vi "readVNAssss.vi"() -> ()   [LabVIEW 2020]
uses:
  <vilib>/Utility/file.llb/Read Delimited Spreadsheet (DBL).vi
  <vilib>/Utility/file.llb/Write Delimited Spreadsheet (string).vi
panel:
  out "all rows 2":dbl[][](array[numeric])
  out "text 2":string
  out "after substring 2":string
  out "string array 4":string[](array[string])
  out "string array 3":string[][](array[string])
  out "string array 2":string[][](array[string])
  out "string array":string[](array[string])
  out "after substring":string
  out "text":string
  out "all rows":dbl[][](array[numeric])
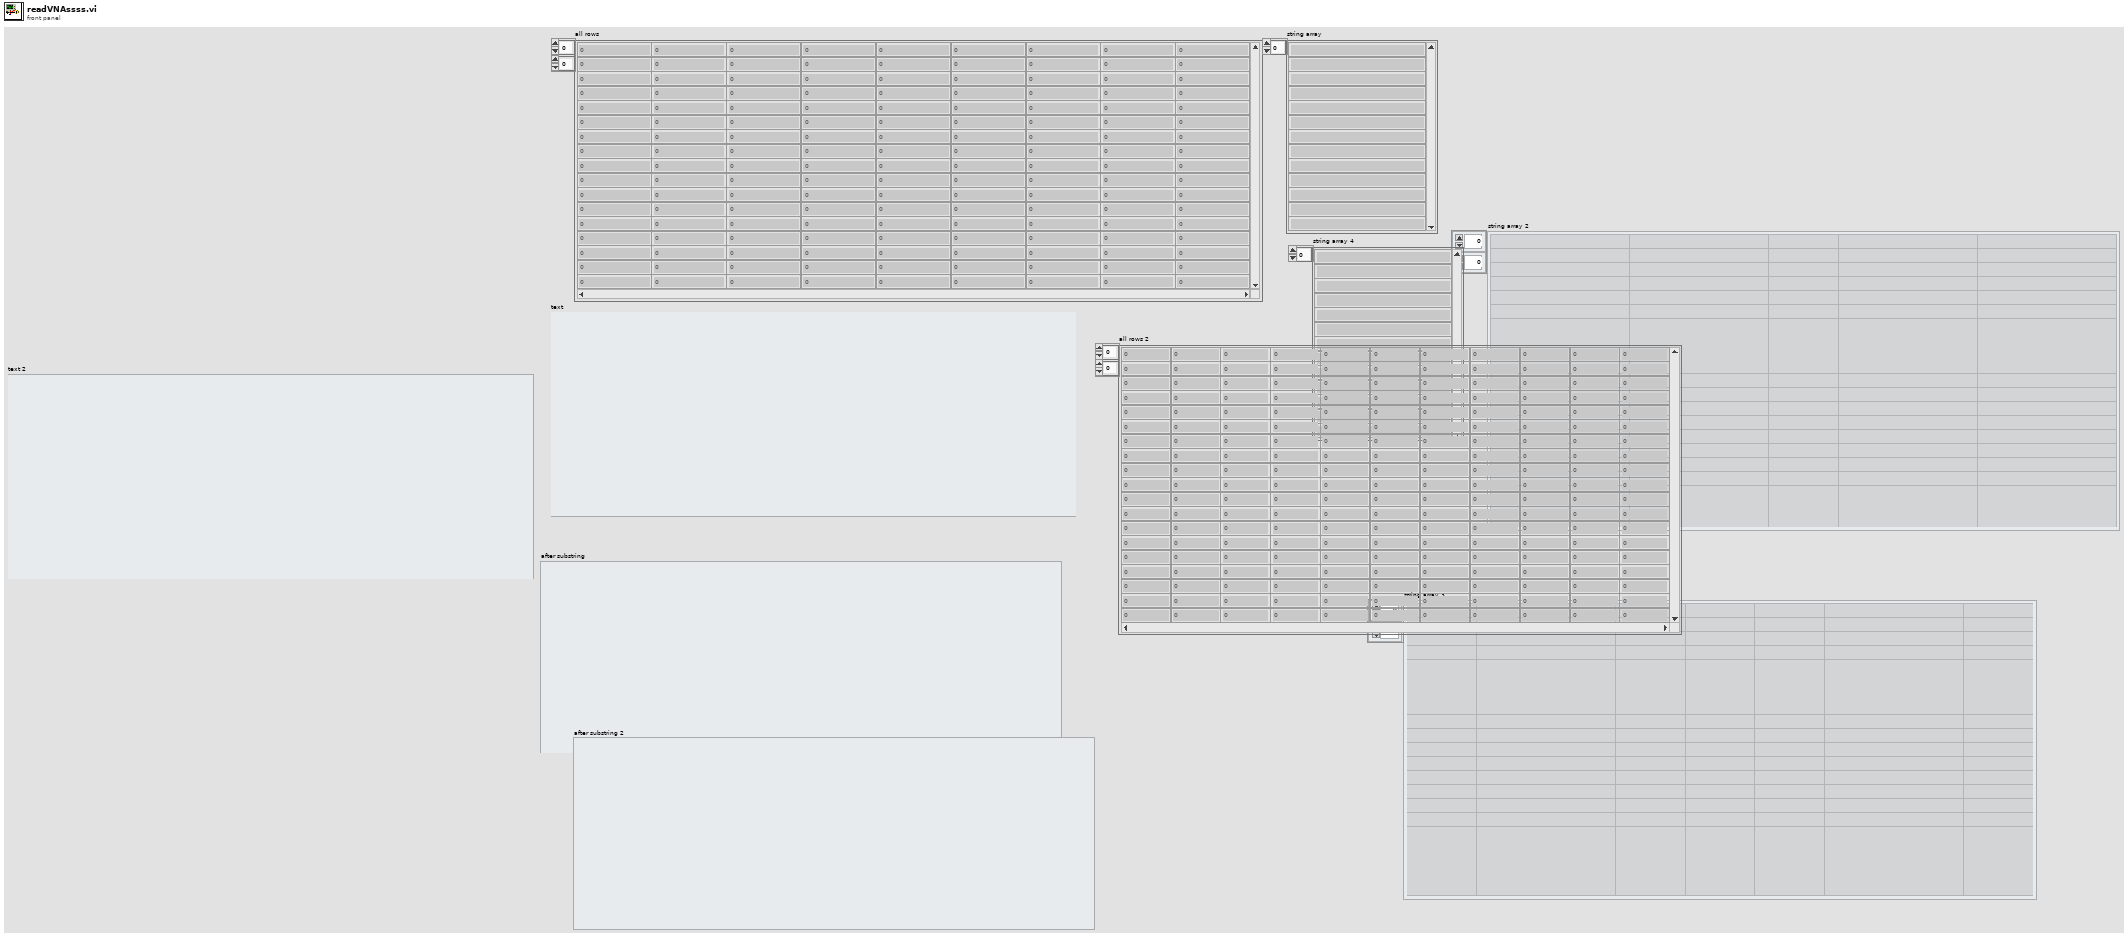
[diagram p1: front panel]
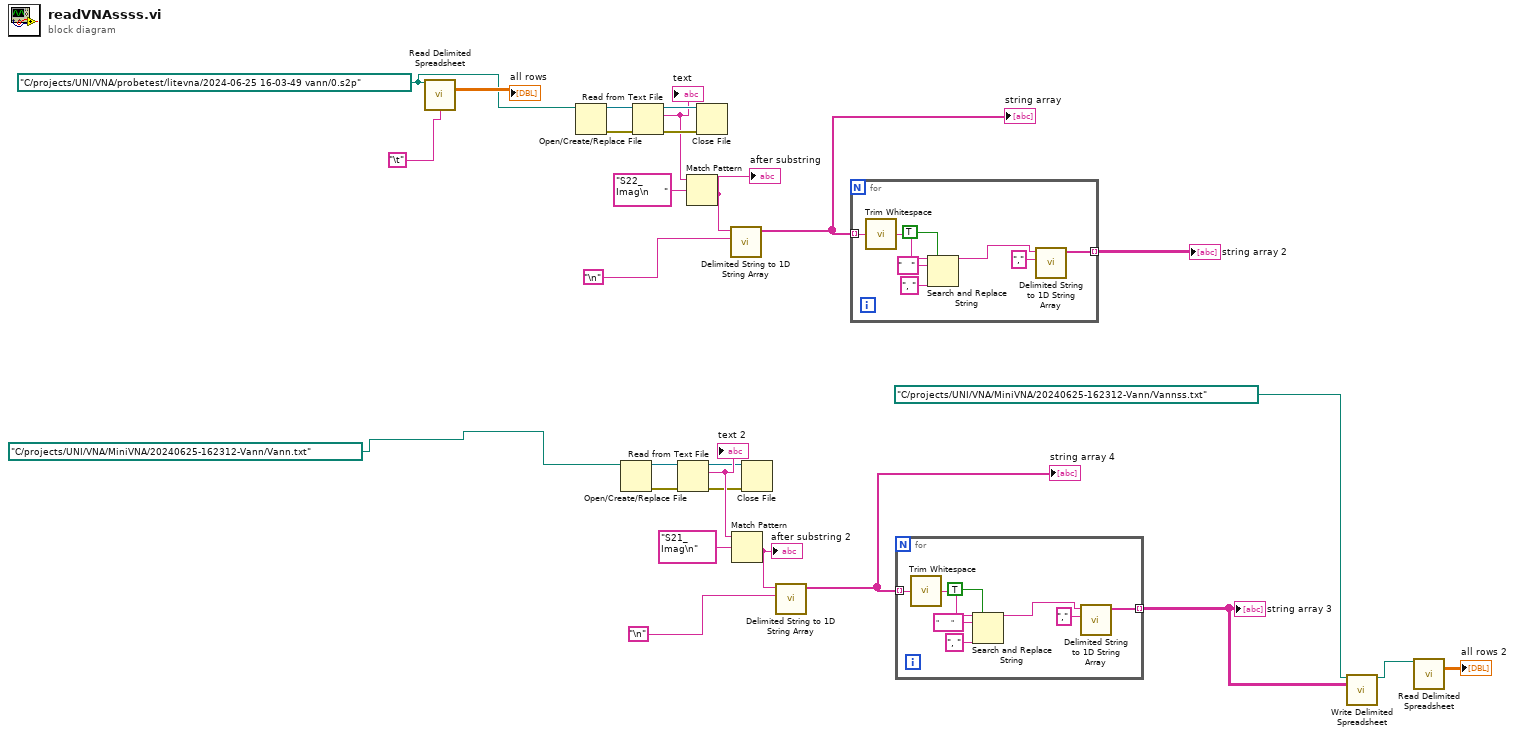
[diagram p0: block diagram]
diagram:
  w21 = path "C:/projects/UNI/VNA/probetest/litevna/2024-06-25 16-03-49 vann/0.s2p" ("file path (dialog if empty)")
  n1 = call-poly <vilib>:"Read Delimited Spreadsheet.vi"("file path (dialog if empty)"=w21, "delimiter (\\t)"="\t") -> ("all rows"=→"all rows":dbl[][])  [unwired: 8 in, 5 out]
  n2 = Open/Create/Replace File(file path (use dialog)=w21) -> (refnum out=w25:refnum<file>, error out=w22:errorcluster)  [unwired: 5 in, 1 out]
  n3 = Open/Create/Replace File(file path (use dialog)=path "C:/projects/UNI/VNA/MiniVNA/20240625-162312-Vann/Vann.txt" ("file path (dialog if empty)")) -> (refnum out=w6:refnum<file>, error out=w9:errorcluster)  [unwired: 5 in, 1 out]
  n4 = Read from Text File(file (use dialog)=w25, error in=w22) -> (refnum out=w24:refnum<file>, text=w20:string, error out=w23:errorcluster)  [unwired: 2 in, 1 out]
  "text" <- w20
  n5 = Read from Text File(file (use dialog)=w6, error in=w9) -> (refnum out=w7:refnum<file>, text=w10:string, error out=w8:errorcluster)  [unwired: 2 in, 1 out]
  "text 2" <- w10
  n6 = Match Pattern(string=w20, regular expression="S22_Imag\n     " ("search string/char (-)")) -> (after substring=w15:string)  [unwired: 1 in, 3 out]
  "after substring" <- w15
  n7 = Close File(refnum=w24, error in=w23) -> ()  [unwired: 2 out]
  n8 = call <vilib>:"Delimited String to 1D String Array.vi"("delimiter"="\n", "delimited string"=w15) -> ("string array"=w17:string[])  [unwired: 9 in]
  "string array" <- w17
  n9 = Match Pattern(string=w10, regular expression="S21_Imag\n" ("search string/char (-)")) -> (after substring=w14:string)  [unwired: 1 in, 3 out]
  "after substring 2" <- w14
  n10 = Close File(refnum=w7, error in=w8) -> ()  [unwired: 2 out]
  n11 = call <vilib>:"Delimited String to 1D String Array.vi"("delimiter"="\n", "delimited string"=w14) -> ("string array"=w13:string[])  [unwired: 9 in]
  "string array 4" <- w13
  n12 = for {
    tunnel: w17 -> [w35] mode=indexing
    tunnel: [w34] -> w16 mode=indexing
    n13 = call <vilib>:"Trim Whitespace.vi"("string"=w35) -> ("trimmed string"=w33:string)  [unwired: 1 in]
    n14 = Search and Replace String(replace all?=TRUE ("replace all? (F)"), input string=w33, search string="   ", replace string=", " ("replace string (\"\")")) -> (result string=w28:string)  [unwired: 4 in, 3 out]
    n15 = call <vilib>:"Delimited String to 1D String Array.vi"("delimiter"=",", "delimited string"=w28) -> ("string array"=w34:string[])  [unwired: 9 in]
  }
  "string array 2" <- w16
  n16 = for {
    tunnel: w13 -> [w43] mode=indexing
    tunnel: [w42] -> w4 mode=indexing
    n17 = call <vilib>:"Trim Whitespace.vi"("string"=w43) -> ("trimmed string"=w41:string)  [unwired: 1 in]
    n18 = Search and Replace String(replace all?=TRUE ("replace all? (F)"), input string=w41, search string="      ", replace string=", " ("replace string (\"\")")) -> (result string=w36:string)  [unwired: 4 in, 3 out]
    n19 = call <vilib>:"Delimited String to 1D String Array.vi"("delimiter"=",", "delimited string"=w36) -> ("string array"=w42:string[])  [unwired: 9 in]
  }
  "string array 3" <- w4
  n20 = call-poly <vilib>:"Write Delimited Spreadsheet.vi"("file path (dialog if empty)"=path "C:/projects/UNI/VNA/MiniVNA/20240625-162312-Vann/Vannss.txt", "2D data"=w4) -> ("new file path (Not A Path if cancelled)"=w2:path)  [unwired: 12 in, 1 out]
  n21 = call-poly <vilib>:"Read Delimited Spreadsheet.vi"("file path (dialog if empty)"=w2) -> ("all rows"=→"all rows 2":dbl[][])  [unwired: 9 in, 5 out]
